vi "ATF_PID_screen_V1.1.vi"() -> ()   [LabVIEW 2022 SP3]
panel:
  out "Countdown Timer (CDT)":dbl format="T%<+%H:%M:%S%3u>t"
  out "Date":timestamp format="%<%d/%m/%Y>T"
  in  "Close":bool
  in  "Screen No":dbl
  out "Indian Standard Time (IST)":timestamp format="%<%H:%M:%S%2u>T"
  out "B_GM_P_04":dbl format="%.2f bar"
  out "B_GM_P_03":dbl format="%.2f bar"
  out "B_GM_P_01":dbl format="%.2f bar"
  out "B_GM_P_02":dbl format="%.2f bar"
  out "B_AT_P_08":dbl format="%.2f bar"
  out "B_AT_P_07":dbl format="%.2f bar"
  out "B_AT_FM_01":dbl format="%.2f Kg/s"
  out "B_AT_FM_02":dbl format="%.2f Kg/s"
  out "B_AT_P_05":dbl format="%.2f bar"
  out "B_AT_P_02":dbl format="%.2f bar"
  out "B_AT_T_02":dbl format="%.2f bar"
  out "B_AT_P_06":dbl format="%.2f bar"
  out "B_AT_P_03":dbl format="%.2f bar"
  out "B_AT_T_03":dbl format="%.2f bar"
  out "B_AT_P_04":dbl format="%.2f bar"
  out "B_AT_T_01":dbl format="%.2f bar"
  out "B_AT_P_01":dbl format="%.2f bar"
  out "B_GN_PV_10_HSS":bool
  out "B_GN_PV_10":bool caption="Boolean"
  out "B_GN_PV_11_HSS":bool
  out "B_GN_PV_11":bool caption="Boolean"
  out "B_AT_PV_05_HSS":bool
  out "B_AT_PV_05":bool caption="Boolean"
  out "B_AT_PV_06_HSS":bool
  out "B_AT_PV_06":bool caption="Boolean"
  out "B_AT_PV_02_HSS":bool
  out "B_AT_PV_02":bool caption="Boolean"
  out "B_AT_PV_03_HSS":bool
  out "B_AT_PV_03":bool caption="Boolean"
  out "B_AT_PV_04_HSS":bool
  out "B_AT_PV_04":bool caption="Boolean"
  out "B_AT_PV_07_HSS":bool
  out "B_AT_PV_07":bool caption="Boolean"
  out "B_AT_PV_01_HSS":bool
  out "B_AT_PV_01":bool caption="Boolean"
  out "B_GN_PV_12_HSS":bool
  out "B_GN_PV_12":bool caption="Boolean"
  out "B_GN_PV_13_HSS":bool
  out "B_GN_PV_13":bool caption="Boolean"
  out "B_GN_PV_14_HSS":bool
  out "B_GN_PV_14":bool caption="Boolean"
  out "B_GN_P_27":dbl format="%.2f bar"
  out "B_GN_P_26":dbl format="%.2f bar"
  out "B_GN_T_02":dbl format="%.2f bar"
  out "B_GN_P_28":dbl format="%.2f bar"
  out "B_GN_P_24":dbl format="%.2f bar"
  out "B_GN_P_25":dbl format="%.2f bar"
  out "B_GN_P_21":dbl format="%.2f bar"
  out "B_GN_P_20":dbl format="%.2f bar"
  out "B_GN_P_16":dbl format="%.2f bar"
  out "B_GN_CV_02":dbl format="%.0f %%"
  out "B_GN_CV_02_HSS":bool
  out "B_GN_CV_02":bool caption="Boolean"
  out "B_GN_P_18":dbl format="%.2f bar"
  out "B_GN_P_17":dbl format="%.2f bar"
  out "B_GN_P_19":dbl format="%.2f bar"
  out "B_GN_P_23":dbl format="%.2f bar"
  out "B_GN_P_22":dbl format="%.2f bar"
  out "B_GN_P_14":dbl format="%.2f bar"
  out "B_GN_P_15":dbl format="%.2f bar"
  # "BSTF P&ID SCREEN"
  # "VERSION 1.0"
  # "Connect to all stage JD and ATF EPV"
  # "Stage Non Cryo Valves Command"
  # "TAF/JD Water Ground Valves Command"
  # "Connect to all ground JD and ATF EPV"
  # "GCH4 Ignitor Purge"
  # "Engine ATF Injector Purge"
  # "ATF Feed Line Purge"
  # "ATF Pump Seal Purge"
  # "Booster Pump Drive"
  # "ATF Seal Purge"
  # "ATF Tank Pressurization"
  # "ATF\n12KL\nTANK"
  # "ATF\nFILL"
  # "GCH4\nSource"
  # "GN2\nSource"
  # "GN2\nVaporisr\nSOurce"
  # "CommonGN2\nSource"
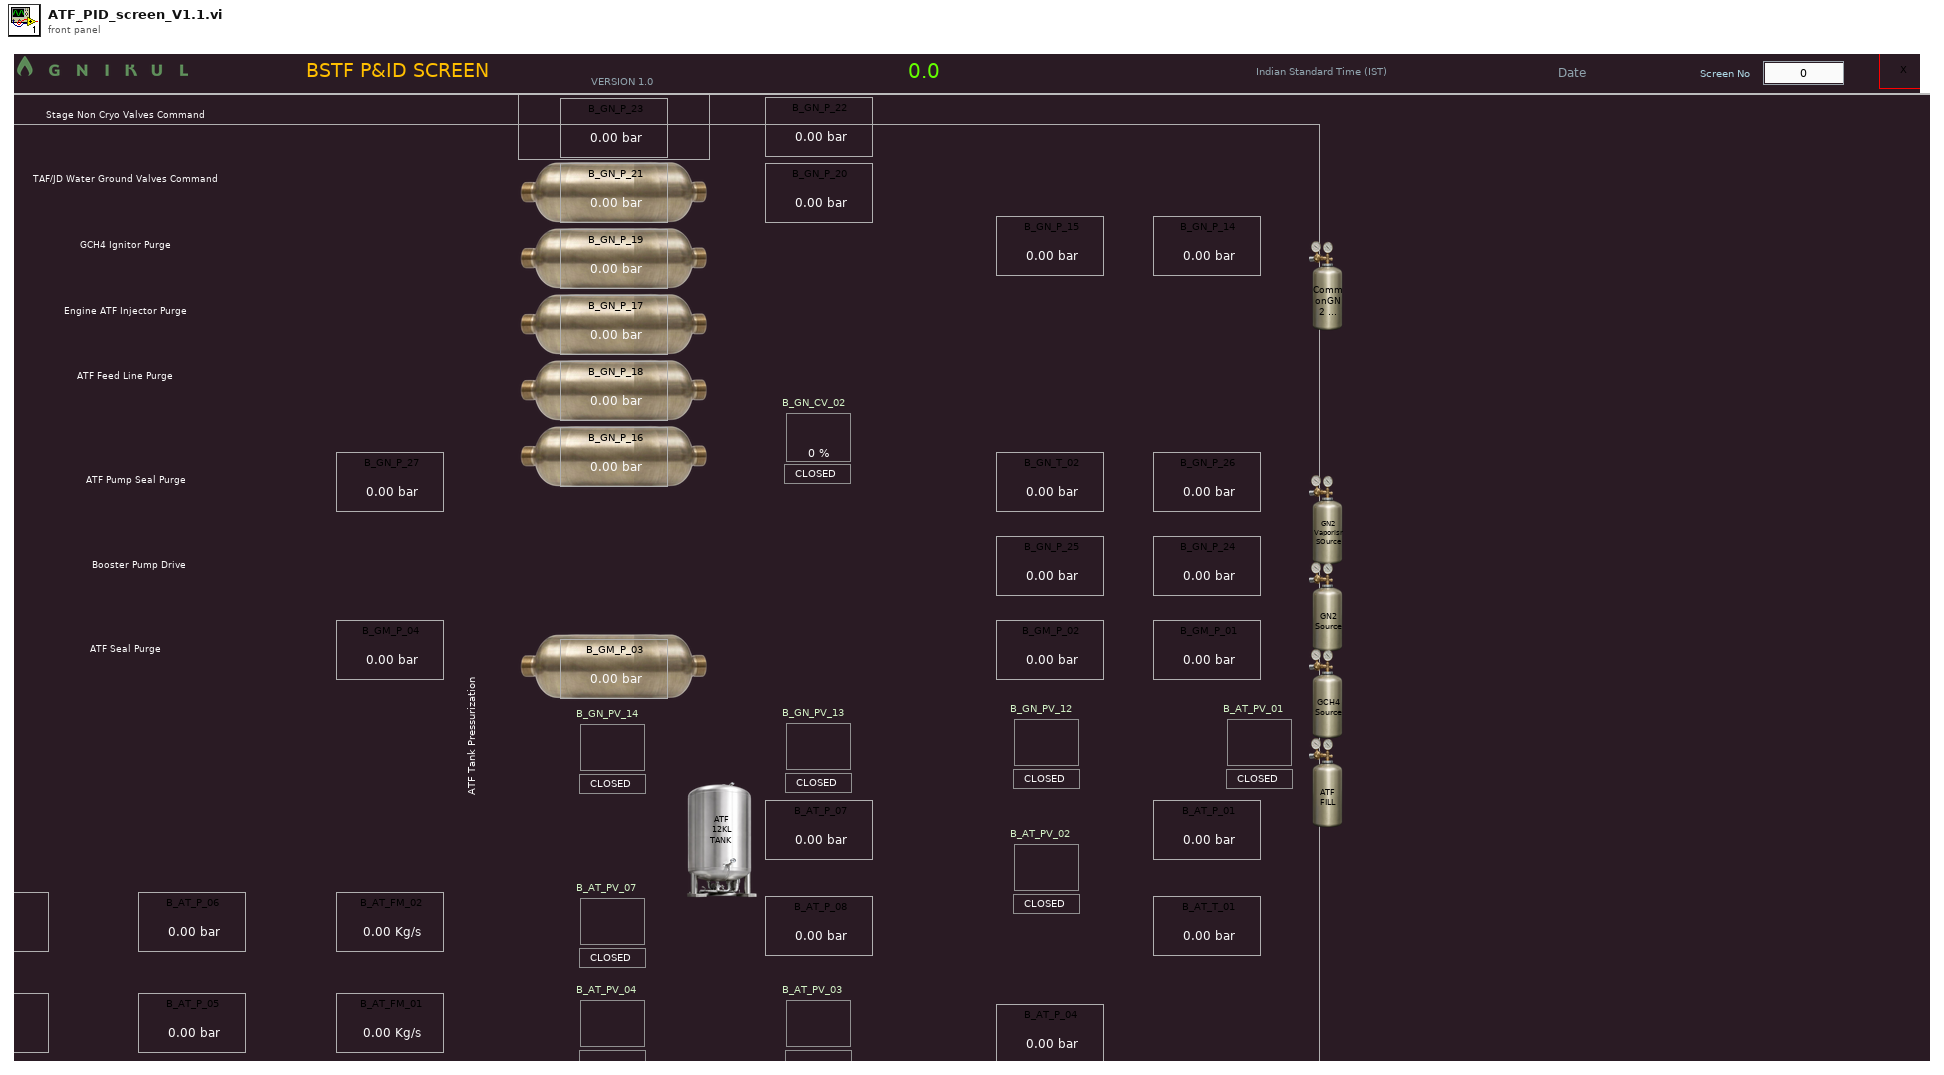
[diagram p1: front panel]
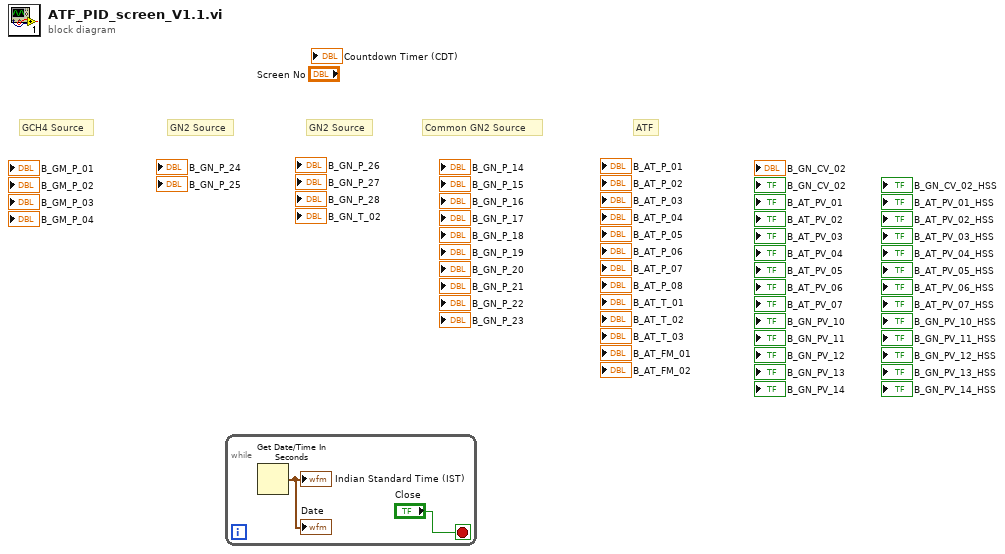
[diagram p0: block diagram]
diagram:
  # "ATF"
  # "Common GN2 Source"
  # "GN2 Source"
  # "GN2 Source"
  # "GCH4 Source"
  n1 = while {
    stop <- "Close" stop-if-true
    n2 = Get Date/Time In Seconds() -> (seconds since 1Jan1904=→"Date" →"Indian Standard Time (IST)":timestamp)
  }
